vi "File_Interface.vi"(6 "Number of byte":i64, 7 "Mode":T1, 8 "에러 입력":errorcluster, 10 "Buffer":string, 11 "Log no":refnum<vi>) -> (0 "error out":errorcluster)   [LabVIEW 2015]
uses:
  File_Control_mode.ctl
  <vilib>/Utility/sysdir.llb/System Directory Type.ctl
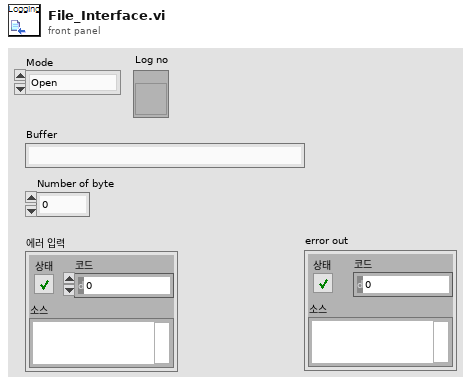
[diagram p1: front panel]
types:
  T1 = typedef "File_Control_mode.ctl" = enum16{"Open", "Write", "Close"}
  T2 = enum8{"Enabled", "Disabled", "Disabled and Grayed Out"}
  T3 = enum16{"open", "replace", "create", "open or create", "replace or create", "replace or create with confirmation"}
  T4 = typedef "System Directory Type.ctl" = i32
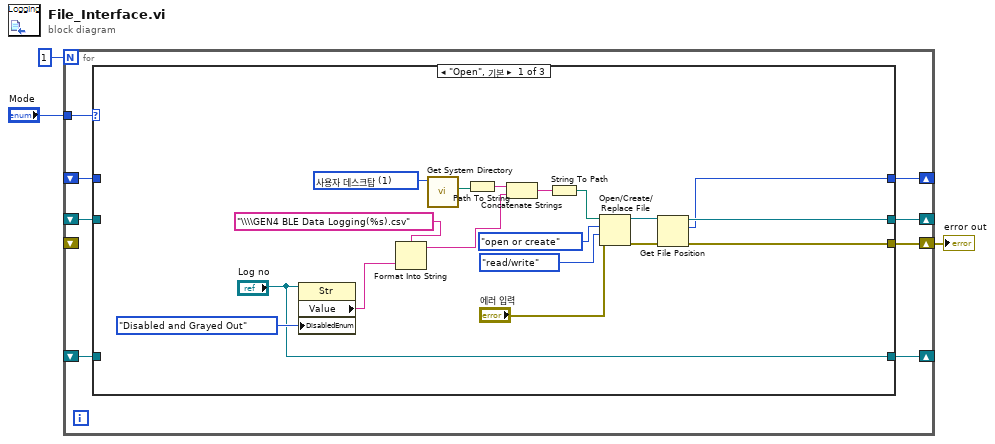
[diagram p0: block diagram]
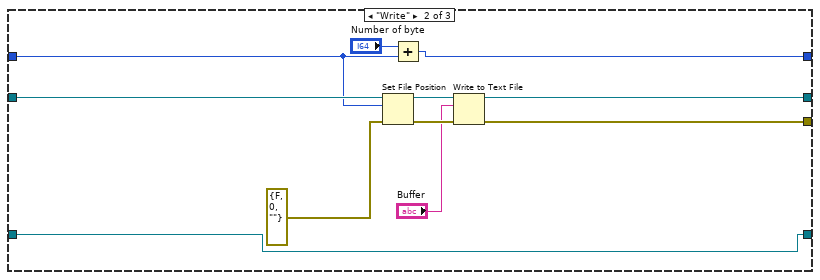
[diagram p2: hidden frame]
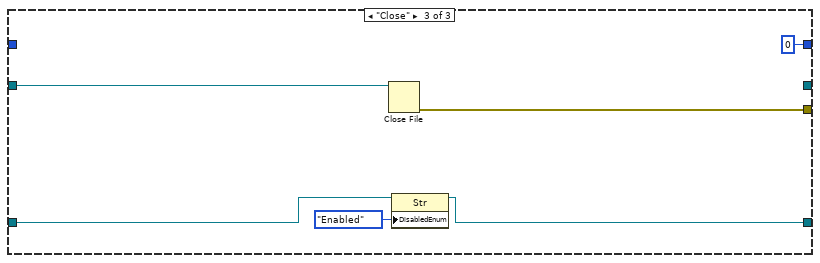
[diagram p3: hidden frame]
diagram:
  n1 = for {
    N: 1 -> [_]
    tunnel: "Mode" -> [w11]
    shift-right: [w10] -> _
    shift-left: _ -> [w7]
    shift-right: [w9] -> w1
    shift-left: _ -> [_]
    shift-right: [w8] -> _
    shift-left: _ -> [w6]
    shift-right: [w5] -> _
    shift-left: _ -> [w4]
    n2 = case shown="\"Open\", 기본" w11 {
      tunnel: [w18 w33 _] -> w10
      tunnel: [w17 w38 w44] -> w9
      tunnel: [w16 w32 i64 0 ("offset (in bytes)")] -> w8
      tunnel: w7 -> [_ w37 w46]
      tunnel: w6 -> [_ w35 _]
      tunnel: ["Log no" w30 w41] -> w5
      tunnel: w4 -> [_ w30 w43]
      frame "Open", Default {
        w27 = T4 1 items=["사용자 홈"=0, "사용자 데스크탑"=1, "사용자 문서"=2, "사용자 어플리케이션 데이터"=3, "사용자 환경"=4, "사용자 임시"=5, "퍼블릭 문서"=6, "퍼블릭 어플리케이션 데이터"=7, "퍼블릭 환경"=8, "퍼블릭 캐시"=13, "시스템 코어 라이브러리"=9, "시스템 설치된 라이브러리"=10, "어플리케이션 파일"=11, "부팅 볼륨 루트"=12] ("system directory type")
        n3 = property class="Str"(reference="Log no", "DisabledEnum"=T2."Disabled and Grayed Out" ("비활성화")) -> ("Value"=w14:string)  [unwired: 1 in, 2 out]
        n4 = Format Into String(format string="\\\\GEN4 BLE Data Logging(%s).csv" ("문자열"), w14) -> (resulting string=w19:string)  [unwired: 2 in, 1 out]
        n5 = call <vilib>:"Get System Directory.vi"("system directory type"=w27) -> ("system directory"=w26:path)  [unwired: 10 in]
        n6 = Path To String(path=w26) -> (string=w25:string)
        n7 = Concatenate Strings(w25, w19) -> (w24:string)
        n8 = String To Path(string=w24) -> (path=w23:path)
        n9 = Open/Create/Replace File(file path (use dialog)=w23, error in="에러 입력", operation (0:open)=T3."open or create" ("동작(0:open)"), access (0:read/write)=enum16{"read/write", "read-only", "write-only"}."read/write" ("접근(0:읽기/쓰기)")) -> (refnum out=w29:refnum<file>, error out=w28:errorcluster)  [unwired: 2 in, 1 out]
        n10 = Get File Position(4:w28, 7:w29) -> (0:w17:errorcluster, 2:w16:i64, 3:w18:refnum<file>)
      }
      frame "Write" {
        n11 = Set File Position(offset (in bytes) (0)=w35, refnum=w37, error in=errorcluster {"status"=FALSE, "code"=0, "source"=""} ("에러 입력")) -> (refnum out=w40:refnum<file>, error out=w39:errorcluster)  [unwired: 1 in]
        n12 = Add(x="Number of byte", y=w35) -> (x+y=w32:i64)
        n13 = Write to Text File(file (use dialog)=w40, text="Buffer", error in=w39) -> (refnum out=w33:refnum<file>, error out=w38:errorcluster)  [unwired: 1 in, 1 out]
      }
      frame "Close" {
        n14 = Close File(refnum=w46) -> (error out=w44:errorcluster)  [unwired: 1 in, 1 out]
        n15 = property class="Str"(reference=w43, "DisabledEnum"=T2."Enabled" ("비활성화")) -> (reference out=w41:refnum<vi>)  [unwired: 1 in, 1 out]
      }
    }
  }
  "error out" <- w1
